vi "CSTK_Icon_Creator_CreateLogo.vi"(8 "错误输入（无错误）":errorcluster, 10 "LOGO输入":u32[][](array[colorbox]), 11 "文件夹路径输入":path) -> (0 "错误输出":errorcluster)   [LabVIEW 2015, in "CSTK_Icon Creator.lvlib"]
uses:
  CSTK_Icon Creator.lvlib
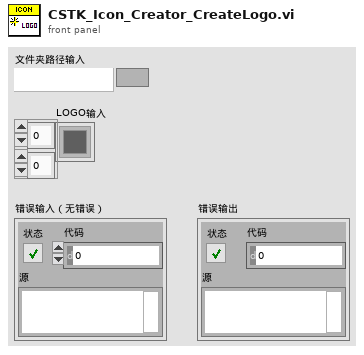
[diagram p1: front panel]
types:
  T1 = typedef "imagedata.ctl" = cluster{"image type":i32, "image depth":i32, "image":u8[], "mask":u8[], "colors":u32[], "Rectangle":cluster{"left":i16, "top":i16, "right":i16, "bottom":i16}}
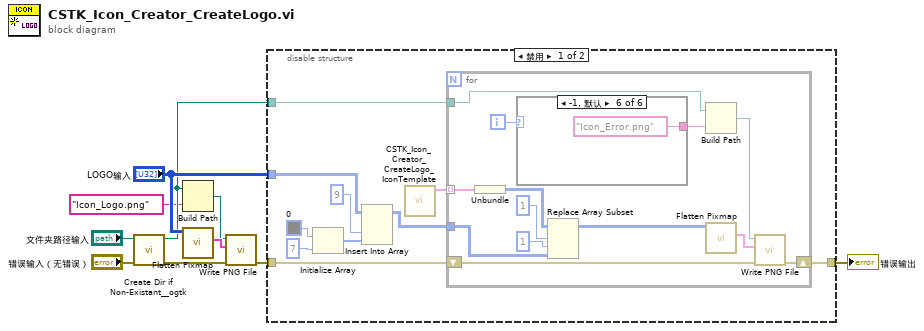
[diagram p0: block diagram]
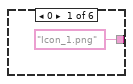
[diagram p2: hidden frame]
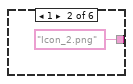
[diagram p3: hidden frame]
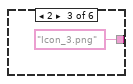
[diagram p4: hidden frame]
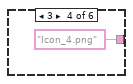
[diagram p5: hidden frame]
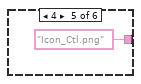
[diagram p6: hidden frame]
diagram:
  n1 = call <userlib>:"Create Dir if Non-Existant__ogtk.vi"("error in (no error)"="错误输入（无错误）", "Directory Path"="文件夹路径输入") -> ("error out"=w2:errorcluster, "dup Directory Path"=w5:path)  [unwired: 7 in, 1 out]
  n2 = Build Path(base path=w5, name or relative path="Icon_Logo.png" ("名称或相对路径")) -> (appended path=w3:path)
  n3 = call <vilib>:"Flatten Pixmap.vi"("24-bit pixmap"="LOGO输入") -> ("image data"=w7:T1)  [unwired: 10 in]
  n4 = call <vilib>:"Write PNG File.vi"("error in (no error)"=w2, "image data"=w7, "path to PNG file"=w3) -> ("error out"=w1:errorcluster)  [unwired: 7 in, 1 out]
  n5 = disable-structure shown="禁用" {
    disable-tunnel: [w19 w40] -> w8
    disable-tunnel: "LOGO输入" -> [w13 _]
    disable-tunnel: w5 -> [w12 _]
    disable-tunnel: w1 -> [w11 w40]
    frame Disabled {
      n6 = Initialize Array(u32 0, 7 ("维数大小")) -> (w14:u32[])
      n7 = Insert Into Array(array=w13, index (col)=9 ("禁用的索引 (列)"), new element=w14) -> (w18:u32[][])  [unwired: 1 in]
      n8 = call "CSTK_Icon_Creator_CreateLogo_IconTemplate.vi"() -> ("Icon Template"=w20:cluster{"Icon_Ctl":u32[][]}[])  [unwired: 11 in]
      n9 = for {
        tunnel: w20 -> [w33] mode=indexing
        tunnel: w18 -> [w29]
        tunnel: w12 -> [w25]
        shift-right: [w22] -> w19
        shift-left: w11 -> [w21]
        i -> [w26]
        n10 = Unbundle(w33) -> ("Icon_Ctl"=w32:u32[][])
        n11 = case shown="-1, 默认" w26 {
          tunnel: ["Icon_1.png" "Icon_2.png" "Icon_3.png" "Icon_4.png" "Icon_Ctl.png" "Icon_Error.png"] -> w24
          frame 0 {
          }
          frame 1 {
          }
          frame 2 {
          }
          frame 3 {
          }
          frame 4 {
          }
          frame -1, Default {
          }
        }
        n12 = Replace Array Subset(array=w32, new element=w29, index (row)=1 ("索引 (行)"), index (col)=1 ("禁用的索引 (列)")) -> (w28:u32[][])
        n13 = Build Path(base path=w25, name or relative path=w24) -> (appended path=w23:path)
        n14 = call <vilib>:"Flatten Pixmap.vi"("24-bit pixmap"=w28) -> ("image data"=w27:T1)  [unwired: 10 in]
        n15 = call <vilib>:"Write PNG File.vi"("error in (no error)"=w21, "image data"=w27, "path to PNG file"=w23) -> ("error out"=w22:errorcluster)  [unwired: 7 in, 1 out]
      }
    }
    frame Enabled {
    }
  }
  "错误输出" <- w8
